vi "Set Panel Queue.vi"(8 "error in (no error)":errorcluster, 10 "Panel Queue":refnum<queue>, 11 "BackStage in":refnum<class "BackStage.lvclass">) -> (0 "error out":errorcluster, 3 "BackStage out":refnum<class "BackStage.lvclass">)   [LabVIEW 2015, in "BackStage.lvclass"]
uses:
  BackStage.lvclass
  BackStage.lvclass/BackStage.ctl
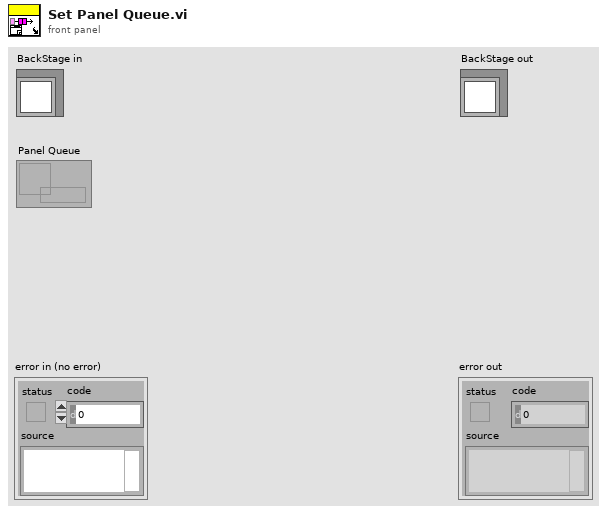
[diagram p1: front panel]
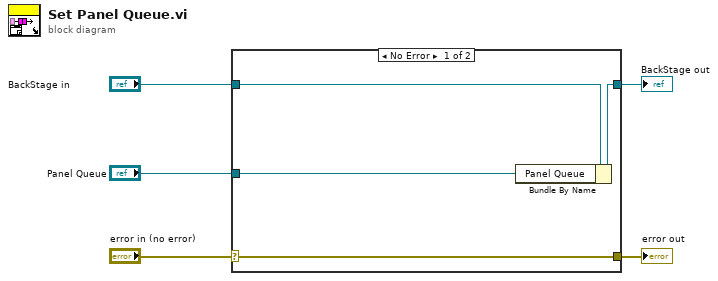
[diagram p0: block diagram]
diagram:
  n1 = case shown="No Error" "error in (no error)" {
    selector: "error in (no error)" -> [w9 w10]
    tunnel: [w9 w10] -> w4
    tunnel: [w7 w11] -> w2
    tunnel: "BackStage in" -> [w8 w11]
    tunnel: "Panel Queue" -> [w6 _]
    frame No Error {
      n2 = Bundle By Name(cluster=w8, "Panel Queue"=w6) -> (w7:refnum<class "BackStage.lvclass">)
    }
    frame Error {
    }
  }
  "error out" <- w4
  "BackStage out" <- w2
